vi "Write Single File Properties.vi"(8 "error in (no error)":errorcluster, 11 "File Properties OUT in":T1) -> (0 "error out":errorcluster, 2 "File Properties OUT out":T1, 3 "VI out":refnum<vi>)   [LabVIEW 2020]
uses:
  TDefs/Single File Properties.ctl
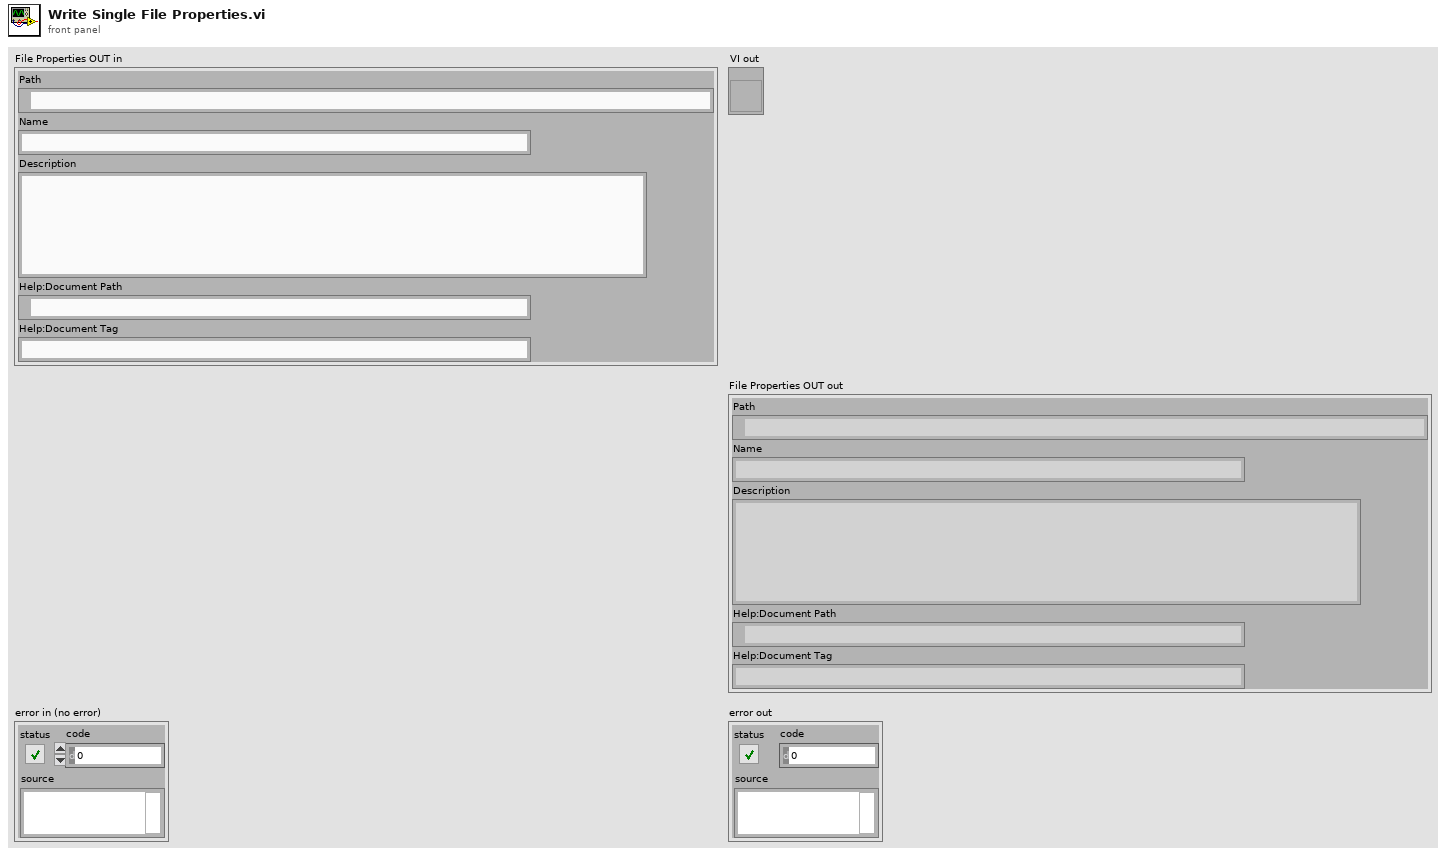
[diagram p1: front panel]
types:
  T1 = typedef "Single File Properties.ctl" = cluster{"Path":path, "Name":string, "Description":string, "Help:Document Path":path, "Help:Document Tag":string}
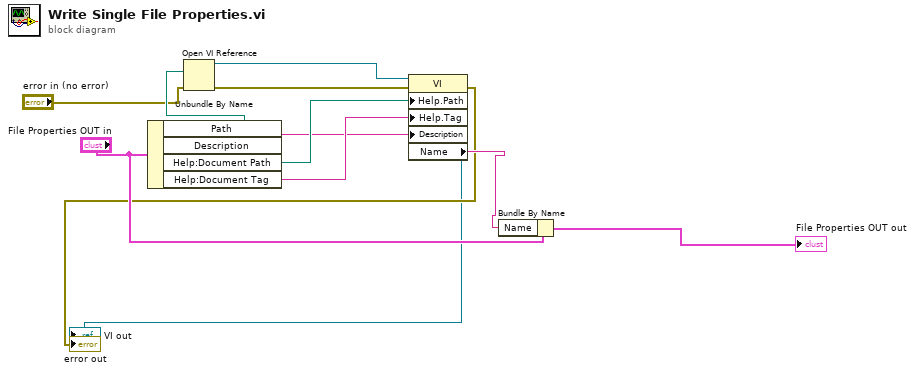
[diagram p0: block diagram]
diagram:
  n1 = Unbundle By Name("File Properties OUT in") -> ("Path"=w6:path, "Description"=w7:string, "Help:Document Path"=w8:path, "Help:Document Tag"=w9:string)
  n2 = Open VI Reference(vi path=w6, error in (no error)="error in (no error)") -> (vi reference=w1:refnum<vi>, error out=w3:errorcluster)  [unwired: 4 in]
  n3 = property class="VI"(reference=w1, error in=w3, "Help.Path"=w8, "Help.Tag"=w9, "Description"=w7) -> (reference out=→"VI out":refnum<vi>, error out=→"error out":errorcluster, "Name"=w10:string)
  n4 = Bundle By Name(cluster="File Properties OUT in", "Name"=w10) -> (→"File Properties OUT out":T1)
